vi "Step to next node.vi"(8 "Numeric":i32, 9 "Nodes":cluster{i32, i32}[](array[cluster]), 10 "Cluster":cluster{i32, i32}, 11 "Grid":bool[][](array[boolean])) -> (3 "Distance to next node":cluster{cluster{i32, i32}, i32}[](array[cluster]))   [LabVIEW 2021]
uses:
  a6cca72e-6f53-4cce-a3df-458a4eb79140.vi
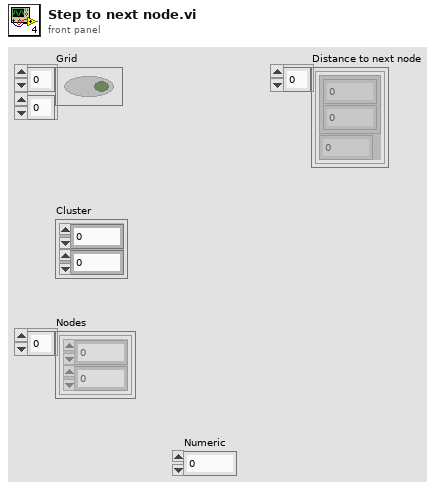
[diagram p1: front panel]
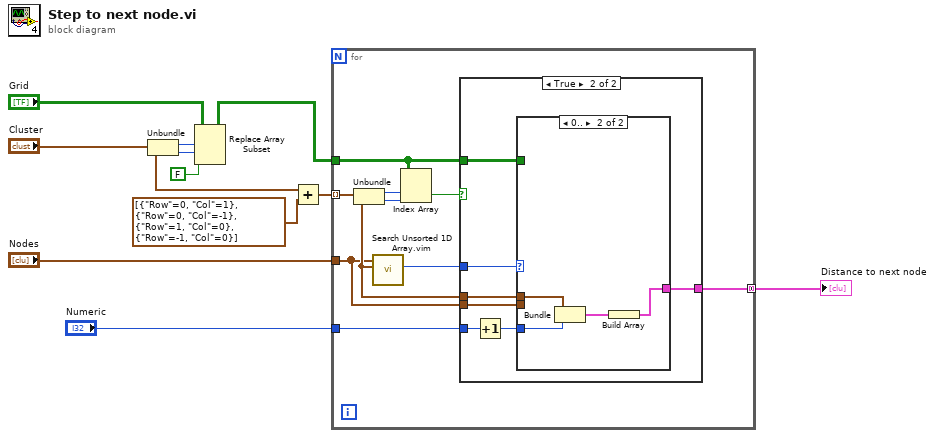
[diagram p0: block diagram]
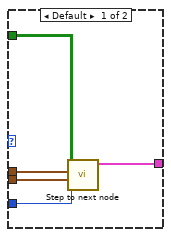
[diagram p3: hidden frame]
diagram:
  n1 = Unbundle("Cluster") -> (w6:i32, w5:i32)
  n2 = Replace Array Subset(array="Grid", new element=FALSE, index (row)=w6, index (col)=w5) -> (w2:bool[][])
  n3 = Add(x="Cluster", y=cluster{"Row":i32, "Col":i32}[] [{"Row"=0, "Col"=1}, {"Row"=0, "Col"=-1}, {"Row"=1, "Col"=0}, {"Row"=-1, "Col"=0}]) -> (x+y=w3:cluster{i32, i32}[])
  n4 = for {
    tunnel: w3 -> [w16] mode=indexing
    tunnel: w2 -> [w13]
    tunnel: "Nodes" -> [w12]
    tunnel: "Numeric" -> [w18]
    tunnel: [w15] -> w11 mode=concatenating
    n5 = Unbundle(w16) -> (w20:i32, w19:i32)
    n6 = call "Search Unsorted 1D Array.vim"("element"=w16, "unsorted 1D array"=w12) -> ("index of element"=w17:i32)  [unwired: 9 in]
    n7 = Index Array(array=w13, index (row)=w20, index (col)=w19) -> (element=w14:bool)
    n8 = case shown="True" w14 {
      tunnel: w18 -> [_ w25]
      tunnel: w17 -> [_ w27]
      tunnel: w16 -> [_ w26]
      tunnel: [_ w23] -> w15
      tunnel: w13 -> [_ w22]
      tunnel: w12 -> [_ w21]
      frame False {
      }
      frame True {
        n9 = Increment(x=w25) -> (x+1=w24:i32)
        n10 = case shown="0.." w27 {
          tunnel: w26 -> [w31 w35]
          tunnel: w24 -> [w30 w36]
          tunnel: [w28 w33] -> w23
          tunnel: w22 -> [w32 _]
          tunnel: w21 -> [w29 _]
          frame Default {
            n11 = call "Step to next node.vi"("Numeric"=w30, "Nodes"=w29, "Cluster"=w31, "Grid"=w32) -> ("Distance to next node"=w28:cluster{cluster{i32, i32}, i32}[])  [unwired: 7 in]
          }
          frame 0.. {
            n12 = Bundle(w35, w36) -> (w34:cluster{cluster{i32, i32}, i32})  [unwired: 1 in]
            n13 = Build Array(w34) -> (w33:cluster{cluster{i32, i32}, i32}[])
          }
        }
      }
    }
  }
  "Distance to next node" <- w11
